vi "Test ON OFF TESynC GUI.vi"() -> ()   [LabVIEW 2009]
panel:
  in  "Event 6 ON":bool
  in  "Event 6 OFF":bool
  out "Event 6":bool
  in  "Event 5 ON":bool
  in  "Event 5 OFF":bool
  out "Event 5":bool
  in  "Event 4 ON":bool
  in  "Event 4 OFF":bool
  out "Event 4":bool
  in  "Event 3 ON":bool
  in  "Event 3 OFF":bool
  out "Event 3":bool
  in  "Event 2 ON":bool
  in  "Event 2 OFF":bool
  out "Event 2":bool
  in  "Event 1 ON":bool
  in  "Event 1 OFF":bool
  out "Event 1":bool
  in  "Chamber On":bool
  in  "Chamber Off":bool
  out "Chamber ON/OFF LED":bool
  in  "Interface\nType":refnum<visa-resource-name>
  in  "ClearErrors":bool
  in  "AlarmAck":bool
  out "Alarm":string
  out "Errors":string
  in  "stop":bool
  out "Actual Humid":dbl format="%.1f"
  in  "SetPoint Humid":dbl format="%.1f"
  out "Actual Temp":dbl format="%.1f"
  in  "SetPoint Temp":dbl format="%.1f"
  in  "error in (no error)":errorcluster
  # "Tidal Engineering Control Panel"
  # "Chan. 2 - Humidity (% RH)"
  # "Chamber State"
  # "Set \nPoint"
  # "Actual"
  # "EVENTS"
  # "STATUS"
  # "www.TidalEngineering.com"
  # "Ver. TESynC 1.1"
  # "Chan. 1 - Temp (deg C)"
  # "Set \nPoint"
  # "Actual"
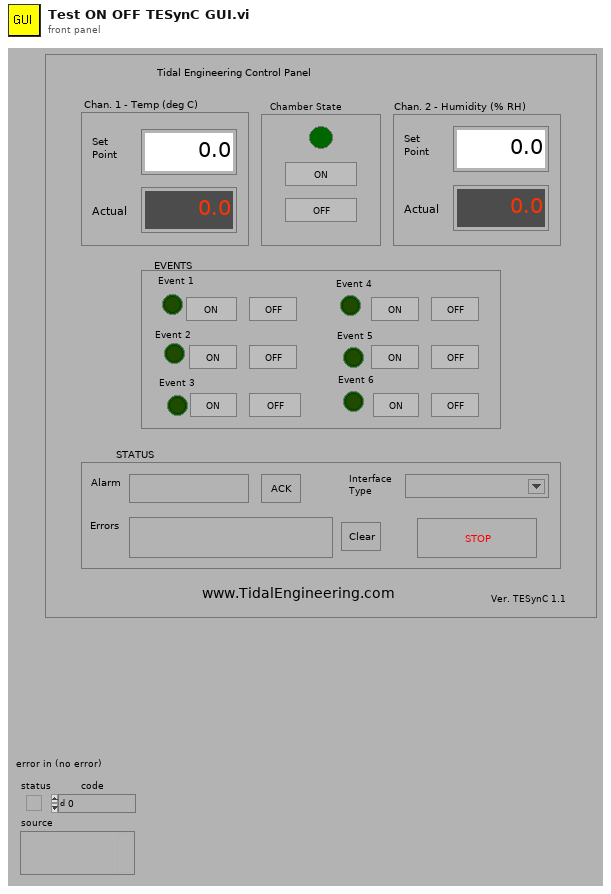
[diagram p1: front panel]
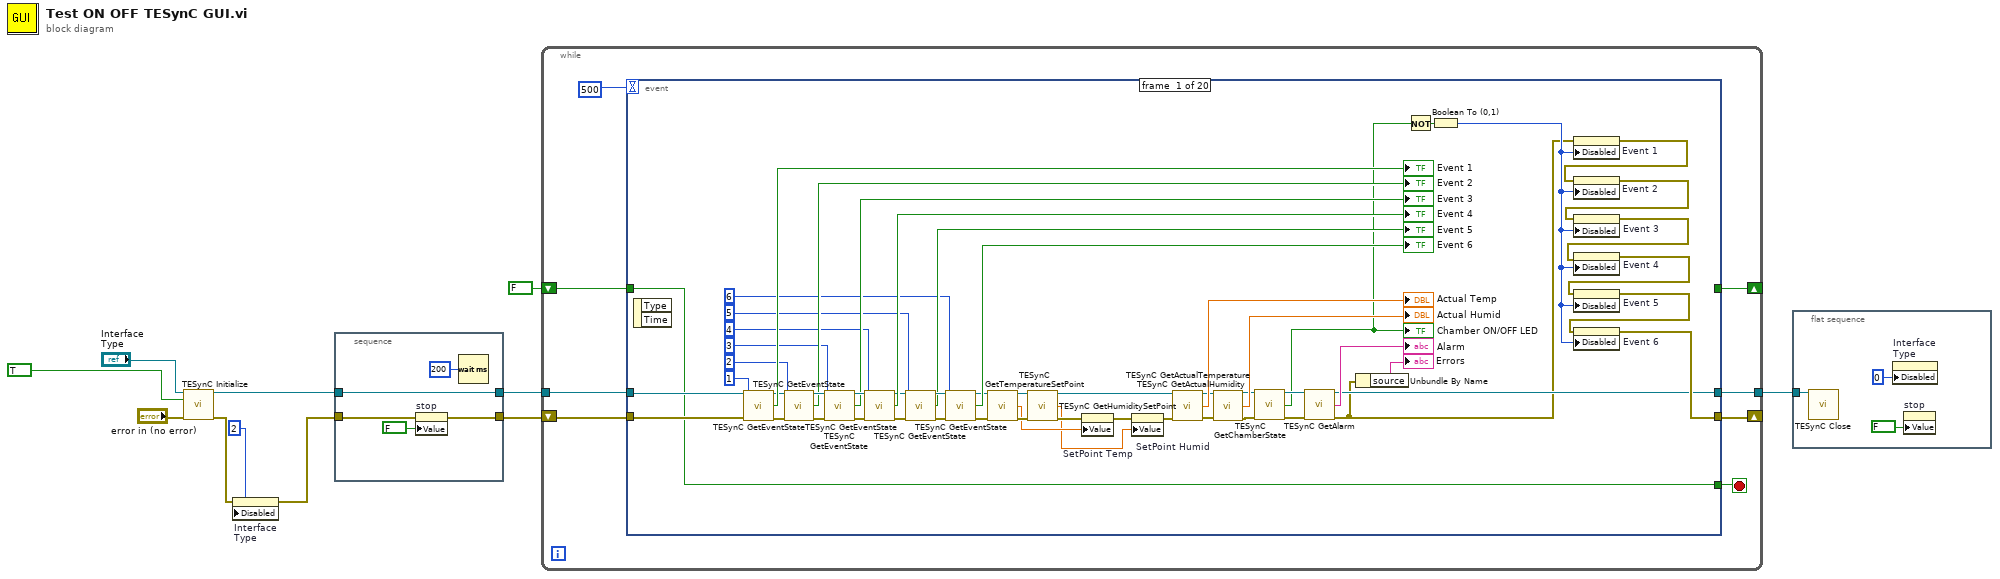
[diagram p0: block diagram]
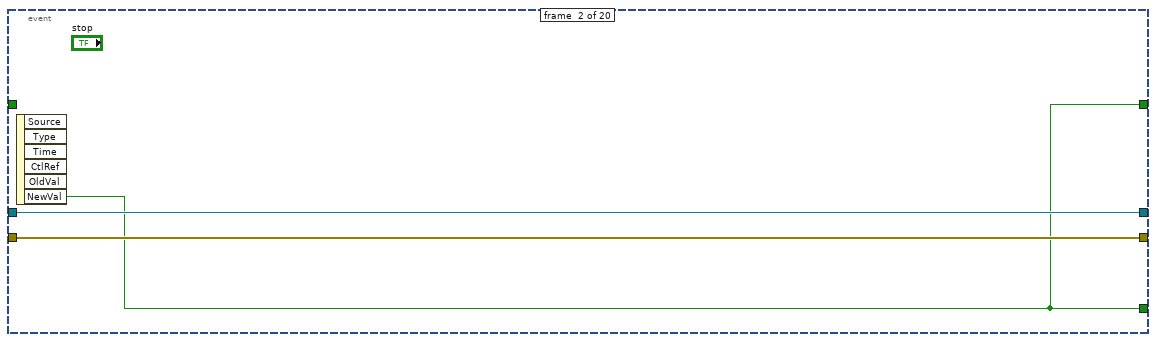
[diagram p2: hidden frame]
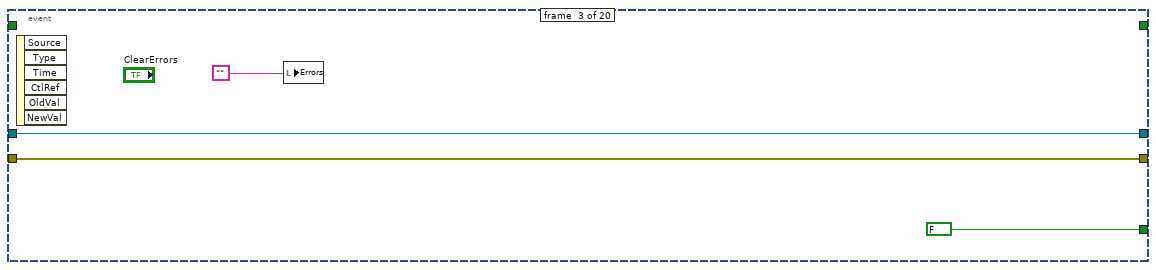
[diagram p3: hidden frame]
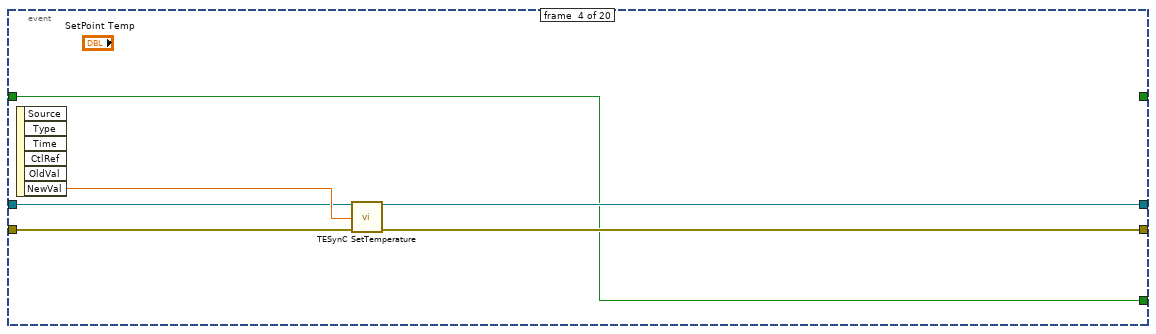
[diagram p4: hidden frame]
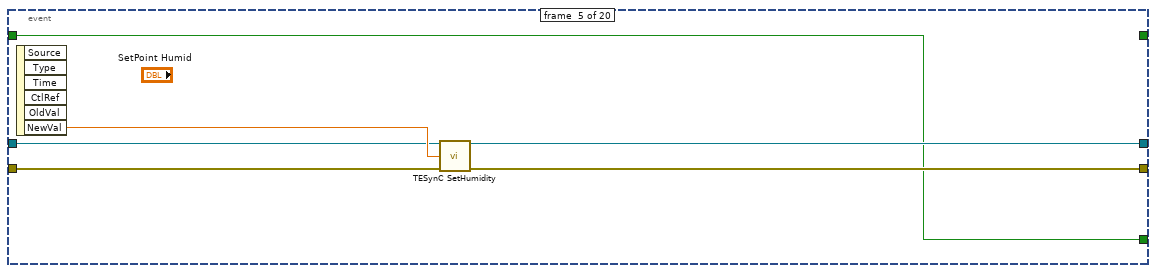
[diagram p5: hidden frame]
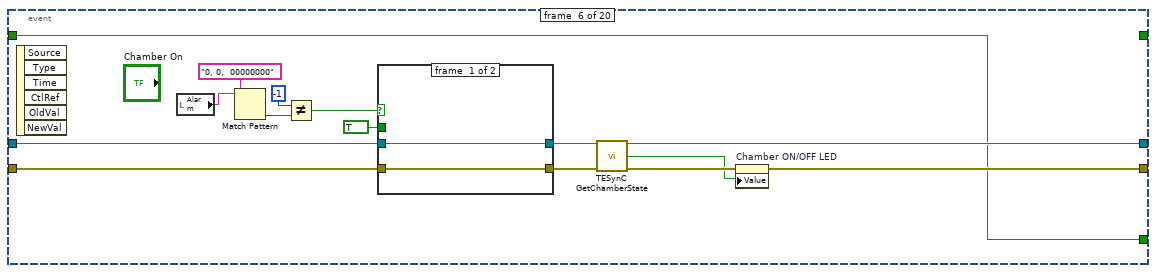
[diagram p6: hidden frame]
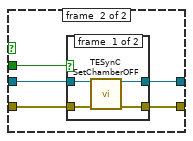
[diagram p7: hidden frame]
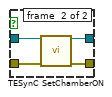
[diagram p8: hidden frame]
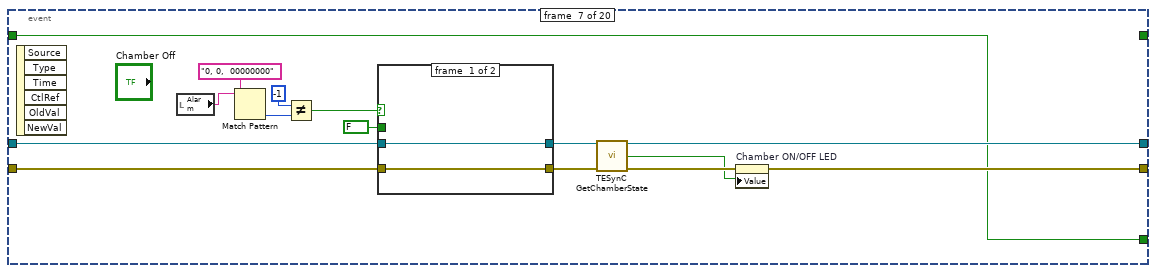
[diagram p9: hidden frame]
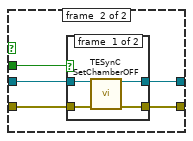
[diagram p10: hidden frame]
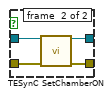
[diagram p11: hidden frame]
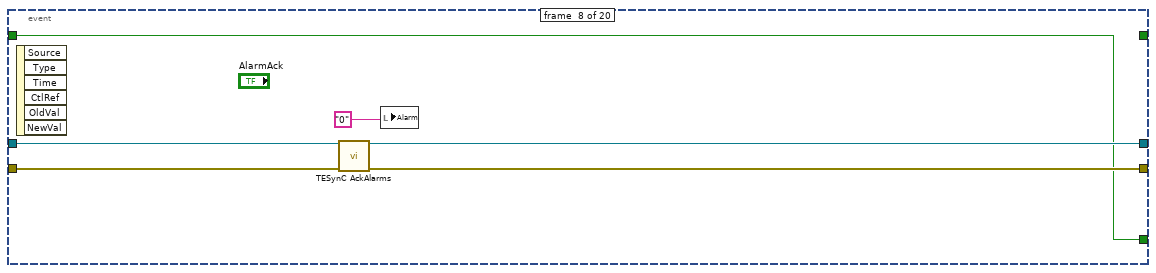
[diagram p12: hidden frame]
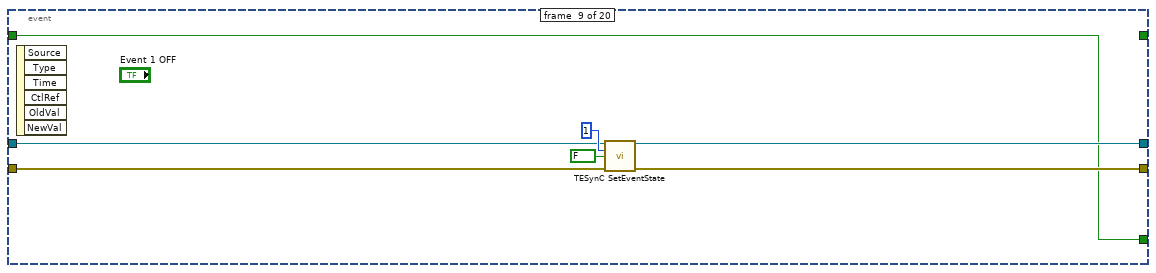
[diagram p13: hidden frame]
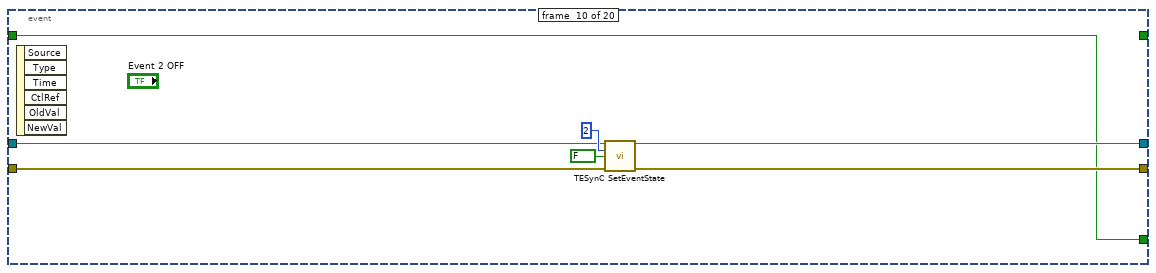
[diagram p14: hidden frame]
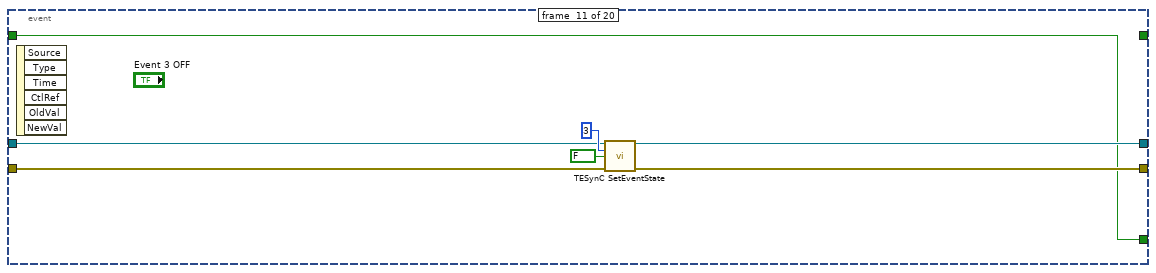
[diagram p15: hidden frame]
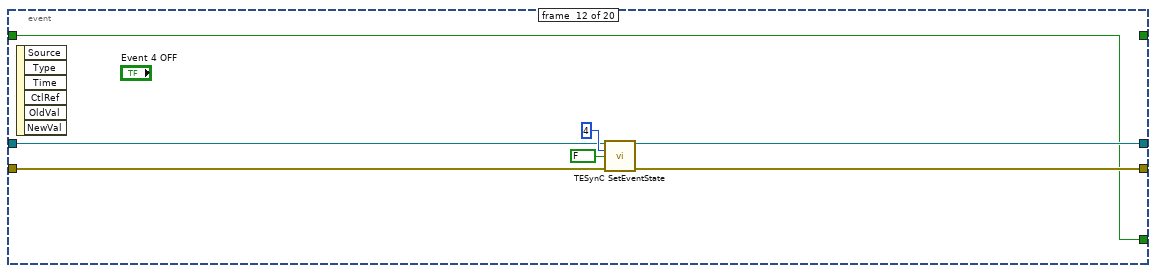
[diagram p16: hidden frame]
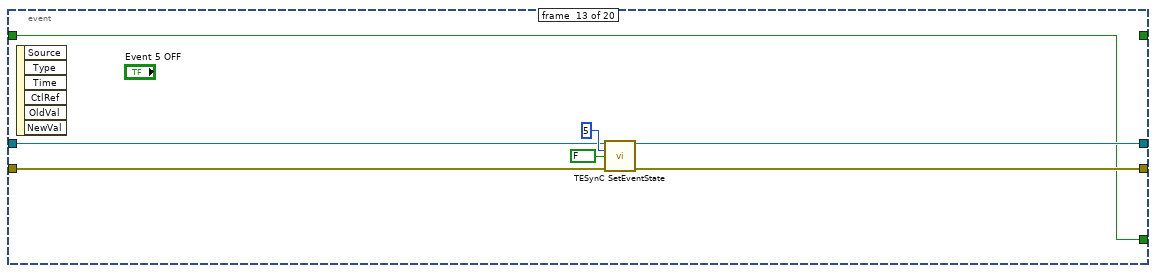
[diagram p17: hidden frame]
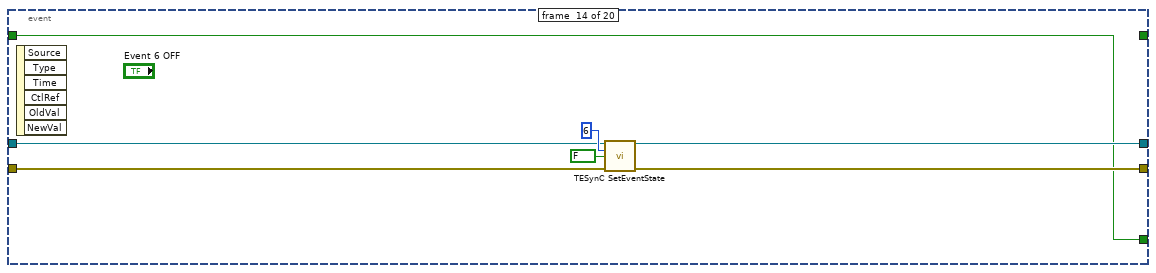
[diagram p18: hidden frame]
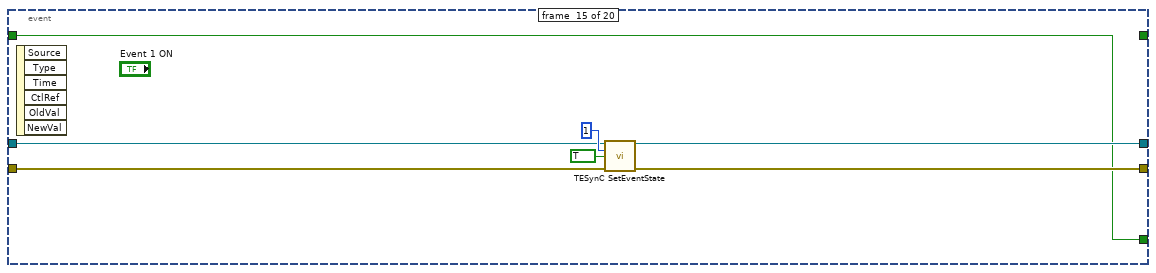
[diagram p19: hidden frame]
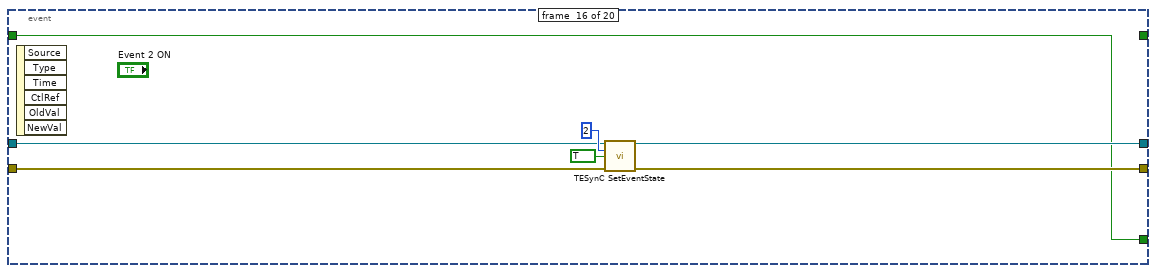
[diagram p20: hidden frame]
diagram:
  n1 = call "TESynC Initialize.vi"("VISA resource name"="Interface\nType", "ID Query (T: Check)"=TRUE, "error in (no error)"="error in (no error)") -> ("VISA session"=w10:refnum<visa-resource-name>, "error out"=w3:errorcluster)  [unwired: 11 in]
  n2 = property on="Interface\nType" class="VISAName"(error in=w3, "Disabled"=u8 2) -> (error out=w2:errorcluster)  [unwired: 1 in, 1 out]
  n3 = stacked-sequence {
    tunnel: [w12] -> w7
    tunnel: w2 -> [w13]
    tunnel: [w16] -> w8
    tunnel: w10 -> [w16]
    frame #0 {
      n4 = property on="stop" class="Bool (strict)"(error in=w13, "Value"=FALSE ("stop")) -> (error out=w12:errorcluster)  [unwired: 1 in, 1 out]
      n5 = Wait (ms)(milliseconds to wait=u32 200) -> ()  [unwired: 1 out]
    }
  }
  n6 = while {
    shift-right: [w21] -> _
    shift-left: w7 -> [w22]
    tunnel: w8 -> [w23]
    tunnel: [w20] -> w9
    shift-right: [w18] -> _
    shift-left: FALSE ("NewVal") -> [w17]
    stop <- w19 stop-if-true
    n7 = event shown="[5] \"Chamber On\": Value Change" {
      selector: _ -> [_ _ _ _ _ _ _ _ _ _ _ _ _ _ _ _ _ _ _ _]
      dyn-events: _ -> [_ _ _ _ _ _ _ _ _ _ _ _ _ _ _ _ _ _ _ _]
      timeout: 500 -> [_ _ _ _ _ _ _ _ _ _ _ _ _ _ _ _ _ _ _ _]
      tunnel: w23 -> [w26 w82 w85 w91 w96 w108 w138 w161 w167 w174 w181 w188 w195 w202 w209 w216 w223 w230 w237 w244]
      tunnel: w22 -> [w28 w83 w86 w93 w99 w109 w139 w165 w172 w179 w186 w193 w200 w207 w214 w221 w228 w235 w242 w249]
      tunnel: [w42 w83 w86 w90 w98 w103 w133 w163 w169 w176 w183 w190 w197 w204 w211 w218 w225 w232 w239 w246] -> w21
      tunnel: [w40 w82 w85 w89 w95 w102 w132 w162 w168 w175 w182 w189 w196 w203 w210 w217 w224 w231 w238 w245] -> w20
      tunnel: [w25 w81 FALSE ("stop") w88 w94 w100 w130 w160 w166 w173 w180 w187 w194 w201 w208 w215 w222 w229 w236 w243] -> w19
      tunnel: [_ w81 _ _ _ _ _ _ _ _ _ _ _ _ _ _ _ _ _ _] -> w18
      tunnel: w17 -> [w25 _ _ w88 w94 w100 w130 w160 w166 w173 w180 w187 w194 w201 w208 w215 w222 w229 w236 w243]
      event #0 {
        n8 = event-data() -> ()  [unwired: 1 in, 2 out]
        n9 = call "TESynC GetEventState.vi"("VISA session in"=w26, "Event Number"=u8 1 ("Event number"), "error in (no error)"=w28) -> ("VISA session out"=w73:refnum<visa-resource-name>, "Event State Readback (1=ON,0=OFF)"=→"Event 1":bool, "error out"=w72:errorcluster)  [unwired: 10 in]
        n10 = call "TESynC GetEventState.vi"("VISA session in"=w73, "Event Number"=u8 2 ("Event number"), "error in (no error)"=w72) -> ("VISA session out"=w71:refnum<visa-resource-name>, "Event State Readback (1=ON,0=OFF)"=→"Event 2":bool, "error out"=w70:errorcluster)  [unwired: 10 in]
        n11 = call "TESynC GetEventState.vi"("VISA session in"=w71, "Event Number"=u8 3 ("Event number"), "error in (no error)"=w70) -> ("VISA session out"=w69:refnum<visa-resource-name>, "Event State Readback (1=ON,0=OFF)"=→"Event 3":bool, "error out"=w68:errorcluster)  [unwired: 10 in]
        n12 = call "TESynC GetEventState.vi"("VISA session in"=w69, "Event Number"=u8 4 ("Event number"), "error in (no error)"=w68) -> ("VISA session out"=w55:refnum<visa-resource-name>, "Event State Readback (1=ON,0=OFF)"=→"Event 4":bool, "error out"=w67:errorcluster)  [unwired: 10 in]
        n13 = call "TESynC GetEventState.vi"("VISA session in"=w55, "Event Number"=u8 5 ("Event number"), "error in (no error)"=w67) -> ("VISA session out"=w66:refnum<visa-resource-name>, "Event State Readback (1=ON,0=OFF)"=→"Event 5":bool, "error out"=w65:errorcluster)  [unwired: 10 in]
        n14 = call "TESynC GetEventState.vi"("VISA session in"=w66, "Event Number"=u8 6 ("Event number"), "error in (no error)"=w65) -> ("VISA session out"=w38:refnum<visa-resource-name>, "Event State Readback (1=ON,0=OFF)"=→"Event 6":bool, "error out"=w39:errorcluster)  [unwired: 10 in]
        n15 = call "TESynC GetTemperatureSetPoint.vi"("VISA session in"=w38, "error in (no error)"=w39) -> ("VISA session out"=w37:refnum<visa-resource-name>, "Temp Setpoint Readback (C)"=w31:dbl, "error out"=w36:errorcluster)  [unwired: 11 in]
        n16 = call "TESynC GetHumiditySetPoint.vi"("VISA session in"=w37, "error in (no error)"=w36) -> ("VISA session out"=w35:refnum<visa-resource-name>, "Setpoint Humidity Readback(%)"=w30:dbl, "error out"=w34:errorcluster)  [unwired: 11 in]
        n17 = property on="SetPoint Temp" class="Digital (strict)"(error in=w34, "Value"=w31) -> (error out=w33:errorcluster)  [unwired: 1 in, 1 out]
        n18 = property on="SetPoint Humid" class="Digital (strict)"(error in=w33, "Value"=w30) -> (error out=w32:errorcluster)  [unwired: 1 in, 1 out]
        n19 = call "TESynC GetActualTemperature.vi"("VISA session in"=w35, "error in (no error)"=w32) -> ("VISA session out"=w76:refnum<visa-resource-name>, "Actual Temp Readback (C)"=→"Actual Temp":dbl, "error out"=w75:errorcluster)  [unwired: 11 in]
        n20 = call "TESynC GetActualHumidity.vi"("VISA session in"=w76, "error in (no error)"=w75) -> ("VISA session out"=w78:refnum<visa-resource-name>, "Actual Humidity Readback (%)"=→"Actual Humid":dbl, "error out"=w77:errorcluster)  [unwired: 11 in]
        n21 = call "TESynC GetChamberState.vi"("VISA session in"=w78, "error in (no error)"=w77) -> ("VISA session out"=w51:refnum<visa-resource-name>, "Chamber State Readback (1=ON,0=OFF)"=w29:bool, "error out"=w52:errorcluster)  [unwired: 11 in]
        "Chamber ON/OFF LED" <- w29
        n22 = call "TESynC GetAlarm.vi"("VISA session in"=w51, "error in (no error)"=w52) -> ("VISA session out"=w40:refnum<visa-resource-name>, "Alarms"=→"Alarm":string, "error out"=w27:errorcluster)  [unwired: 11 in]
        n23 = Unbundle By Name(w27) -> ("source"=→"Errors":string)
        n24 = Not(x=w29) -> (.not. x?=w48:bool)
        n25 = Boolean To (0,1)(Boolean=w48) -> (0, 1=w41:i16)
        n26 = property on="Event 1" class="Boolean (strict)"(error in=w27, "Disabled"=w41) -> (error out=w47:errorcluster)  [unwired: 1 in, 1 out]
        n27 = property on="Event 2" class="Boolean (strict)"(error in=w47, "Disabled"=w41) -> (error out=w46:errorcluster)  [unwired: 1 in, 1 out]
        n28 = property on="Event 3" class="Boolean (strict)"(error in=w46, "Disabled"=w41) -> (error out=w45:errorcluster)  [unwired: 1 in, 1 out]
        n29 = property on="Event 4" class="Boolean (strict)"(error in=w45, "Disabled"=w41) -> (error out=w44:errorcluster)  [unwired: 1 in, 1 out]
        n30 = property on="Event 5" class="Boolean (strict)"(error in=w44, "Disabled"=w41) -> (error out=w43:errorcluster)  [unwired: 1 in, 1 out]
        n31 = property on="Event 6" class="Boolean (strict)"(error in=w43, "Disabled"=w41) -> (error out=w42:errorcluster)  [unwired: 1 in, 1 out]
      }
      event #1 {
        n32 = event-data() -> ("NewVal"=w81:bool)  [unwired: 1 in, 5 out]
      }
      event #2 {
        n33 = event-data() -> ()  [unwired: 1 in, 6 out]
        n34 = local write "Errors"("") -> ()
      }
      event #3 {
        n35 = event-data() -> ("NewVal"=w92:dbl)  [unwired: 1 in, 5 out]
        n36 = call "TESynC SetTemperature.vi"("VISA session in"=w91, "Temperature (C"=w92, "error in (no error)"=w93) -> ("VISA session out"=w89:refnum<visa-resource-name>, "error out"=w90:errorcluster)  [unwired: 11 in]
      }
      event #4 {
        n37 = event-data() -> ("NewVal"=w97:dbl)  [unwired: 1 in, 5 out]
        n38 = call "TESynC SetHumidity.vi"("VISA session in"=w96, "Humidity (%)"=w97, "error in (no error)"=w99) -> ("VISA session out"=w95:refnum<visa-resource-name>, "error out"=w98:errorcluster)  [unwired: 11 in]
      }
      event #5 {
        n39 = event-data() -> ()  [unwired: 1 in, 6 out]
        n40 = local read "Alarm"() -> (w112:string)
        n41 = Match Pattern(string=w112, regular expression="0, 0,  00000000") -> (offset past match=w113:i32)  [unwired: 1 in, 3 out]
        n42 = Not Equal?(x=-1, y=w113) -> (x != y?=w110:bool)
        n43 = case shown="True" w110 {
          tunnel: w109 -> [w116 w121]
          tunnel: w108 -> [w115 w120]
          tunnel: [w116 w119] -> w107
          tunnel: TRUE ("NewVal") -> [_ w118]
          tunnel: [w115 w117] -> w106
          frame #0 {
          }
          frame #1 {
            n44 = case shown="True" w118 {
              tunnel: w121 -> [w125 w129]
              tunnel: w120 -> [w122 w128]
              tunnel: [w123 w127] -> w117
              tunnel: [w124 w126] -> w119
              frame #0 {
                n45 = call "TESynC SetChamberOFF.vi"("VISA session in"=w122, "error in (no error)"=w125) -> ("VISA session out"=w123:refnum<visa-resource-name>, "error out"=w124:errorcluster)  [unwired: 12 in]
              }
              frame #1 {
                n46 = call "TESynC SetChamberON.vi"("VISA session in"=w128, "error in (no error)"=w129) -> ("VISA session out"=w127:refnum<visa-resource-name>, "error out"=w126:errorcluster)  [unwired: 12 in]
              }
            }
          }
        }
        n47 = call "TESynC GetChamberState.vi"("VISA session in"=w106, "error in (no error)"=w107) -> ("VISA session out"=w102:refnum<visa-resource-name>, "Chamber State Readback (1=ON,0=OFF)"=w104:bool, "error out"=w105:errorcluster)  [unwired: 11 in]
        n48 = property on="Chamber ON/OFF LED" class="Boolean (strict)"(error in=w105, "Value"=w104) -> (error out=w103:errorcluster)  [unwired: 1 in, 1 out]
      }
      event #6 {
        n49 = event-data() -> ()  [unwired: 1 in, 6 out]
        n50 = local read "Alarm"() -> (w142:string)
        n51 = Match Pattern(string=w142, regular expression="0, 0,  00000000") -> (offset past match=w143:i32)  [unwired: 1 in, 3 out]
        n52 = Not Equal?(x=-1, y=w143) -> (x != y?=w140:bool)
        n53 = case shown="True" w140 {
          tunnel: w139 -> [w146 w151]
          tunnel: w138 -> [w145 w150]
          tunnel: [w146 w149] -> w137
          tunnel: FALSE ("NewVal") -> [_ w148]
          tunnel: [w145 w147] -> w136
          frame #0 {
          }
          frame #1 {
            n54 = case shown="True" w148 {
              tunnel: w151 -> [w155 w159]
              tunnel: w150 -> [w152 w158]
              tunnel: [w153 w157] -> w147
              tunnel: [w154 w156] -> w149
              frame #0 {
                n55 = call "TESynC SetChamberOFF.vi"("VISA session in"=w152, "error in (no error)"=w155) -> ("VISA session out"=w153:refnum<visa-resource-name>, "error out"=w154:errorcluster)  [unwired: 12 in]
              }
              frame #1 {
                n56 = call "TESynC SetChamberON.vi"("VISA session in"=w158, "error in (no error)"=w159) -> ("VISA session out"=w157:refnum<visa-resource-name>, "error out"=w156:errorcluster)  [unwired: 12 in]
              }
            }
          }
        }
        n57 = call "TESynC GetChamberState.vi"("VISA session in"=w136, "error in (no error)"=w137) -> ("VISA session out"=w132:refnum<visa-resource-name>, "Chamber State Readback (1=ON,0=OFF)"=w134:bool, "error out"=w135:errorcluster)  [unwired: 11 in]
        n58 = property on="Chamber ON/OFF LED" class="Boolean (strict)"(error in=w135, "Value"=w134) -> (error out=w133:errorcluster)  [unwired: 1 in, 1 out]
      }
      event #7 {
        n59 = event-data() -> ()  [unwired: 1 in, 6 out]
        n60 = call "TESynC AckAlarms.vi"("VISA session in"=w161, "error in (no error)"=w165) -> ("VISA session out"=w162:refnum<visa-resource-name>, "error out"=w163:errorcluster)  [unwired: 12 in]
        n61 = local write "Alarm"("0") -> ()
      }
      event #8 {
        n62 = event-data() -> ()  [unwired: 1 in, 6 out]
        n63 = call "TESynC SetEventState.vi"("VISA session in"=w167, "Event number"=u8 1, "Event State"=FALSE, "error in (no error)"=w172) -> ("VISA session out"=w168:refnum<visa-resource-name>, "error out"=w169:errorcluster)  [unwired: 10 in]
      }
      event #9 {
        n64 = event-data() -> ()  [unwired: 1 in, 6 out]
        n65 = call "TESynC SetEventState.vi"("VISA session in"=w174, "Event number"=u8 2, "Event State"=FALSE, "error in (no error)"=w179) -> ("VISA session out"=w175:refnum<visa-resource-name>, "error out"=w176:errorcluster)  [unwired: 10 in]
      }
      event #10 {
        n66 = event-data() -> ()  [unwired: 1 in, 6 out]
        n67 = call "TESynC SetEventState.vi"("VISA session in"=w181, "Event number"=u8 3, "Event State"=FALSE, "error in (no error)"=w186) -> ("VISA session out"=w182:refnum<visa-resource-name>, "error out"=w183:errorcluster)  [unwired: 10 in]
      }
      event #11 {
        n68 = event-data() -> ()  [unwired: 1 in, 6 out]
        n69 = call "TESynC SetEventState.vi"("VISA session in"=w188, "Event number"=u8 4, "Event State"=FALSE, "error in (no error)"=w193) -> ("VISA session out"=w189:refnum<visa-resource-name>, "error out"=w190:errorcluster)  [unwired: 10 in]
      }
      event #12 {
        n70 = event-data() -> ()  [unwired: 1 in, 6 out]
        n71 = call "TESynC SetEventState.vi"("VISA session in"=w195, "Event number"=u8 5, "Event State"=FALSE, "error in (no error)"=w200) -> ("VISA session out"=w196:refnum<visa-resource-name>, "error out"=w197:errorcluster)  [unwired: 10 in]
      }
      event #13 {
        n72 = event-data() -> ()  [unwired: 1 in, 6 out]
        n73 = call "TESynC SetEventState.vi"("VISA session in"=w202, "Event number"=u8 6, "Event State"=FALSE, "error in (no error)"=w207) -> ("VISA session out"=w203:refnum<visa-resource-name>, "error out"=w204:errorcluster)  [unwired: 10 in]
      }
      event #14 {
        n74 = event-data() -> ()  [unwired: 1 in, 6 out]
        n75 = call "TESynC SetEventState.vi"("VISA session in"=w209, "Event number"=u8 1, "Event State"=TRUE, "error in (no error)"=w214) -> ("VISA session out"=w210:refnum<visa-resource-name>, "error out"=w211:errorcluster)  [unwired: 10 in]
      }
      event #15 {
        n76 = event-data() -> ()  [unwired: 1 in, 6 out]
        n77 = call "TESynC SetEventState.vi"("VISA session in"=w216, "Event number"=u8 2, "Event State"=TRUE, "error in (no error)"=w221) -> ("VISA session out"=w217:refnum<visa-resource-name>, "error out"=w218:errorcluster)  [unwired: 10 in]
      }
      event #16 {
        n78 = event-data() -> ()  [unwired: 1 in, 6 out]
        n79 = call "TESynC SetEventState.vi"("VISA session in"=w223, "Event number"=u8 3, "Event State"=TRUE, "error in (no error)"=w228) -> ("VISA session out"=w224:refnum<visa-resource-name>, "error out"=w225:errorcluster)  [unwired: 10 in]
      }
      event #17 {
        n80 = event-data() -> ()  [unwired: 1 in, 6 out]
        n81 = call "TESynC SetEventState.vi"("VISA session in"=w230, "Event number"=u8 4, "Event State"=TRUE, "error in (no error)"=w235) -> ("VISA session out"=w231:refnum<visa-resource-name>, "error out"=w232:errorcluster)  [unwired: 10 in]
      }
      event #18 {
        n82 = event-data() -> ()  [unwired: 1 in, 6 out]
        n83 = call "TESynC SetEventState.vi"("VISA session in"=w237, "Event number"=u8 5, "Event State"=TRUE, "error in (no error)"=w242) -> ("VISA session out"=w238:refnum<visa-resource-name>, "error out"=w239:errorcluster)  [unwired: 10 in]
      }
      event #19 {
        n84 = event-data() -> ()  [unwired: 1 in, 6 out]
        n85 = call "TESynC SetEventState.vi"("VISA session in"=w244, "Event number"=u8 6, "Event State"=TRUE, "error in (no error)"=w249) -> ("VISA session out"=w245:refnum<visa-resource-name>, "error out"=w246:errorcluster)  [unwired: 10 in]
      }
    }
  }
  n86 = flat-sequence {
    tunnel: w9 -> [w252]
    frame #0 {
      n87 = call "TESynC Close.vi"("VISA session in"=w252) -> ()  [unwired: 14 in, 1 out]
      n88 = property on="Interface\nType" class="VISAName"("Disabled"=u8 0) -> ()  [unwired: 2 in, 2 out]
      n89 = property on="stop" class="Bool (strict)"("Value"=FALSE ("stop")) -> ()  [unwired: 2 in, 2 out]
    }
  }
